vi "AdminLogInGetNoOfTrialsForOneStudent(SubVI).vi"(10 "Admin no":string, 11 "Refnum in":T1) -> (3 "NoOfTrials":i32)   [LabVIEW 2013]
uses:
  <vilib>/addons/database/Connection.llb/Conn ObjectReference.ctl
  <vilib>/addons/database/_DB Variant To Data/Database Variant To Data.xnode
  <vilib>/addons/database/NI_Database_API.lvlib
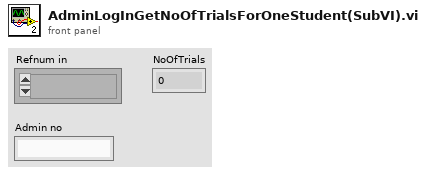
[diagram p1: front panel]
types:
  T1 = typedef "NI_Database_API.lvlib/Conn ObjectReference.ctl" = refnum<k1>
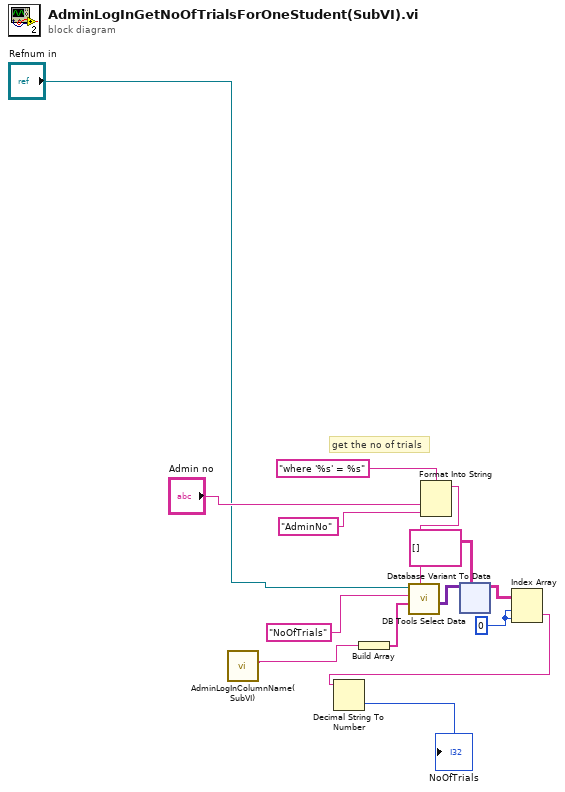
[diagram p0: block diagram]
diagram:
  w8 = 0 ("disabled index (col)")
  # "get the no of trials"
  n1 = call "AdminLogInColumnName(SubVI).vi"() -> ("Path for Score Table"=w1:string)  [unwired: 11 in]
  n2 = Build Array(w1) -> (w5:string[])
  n3 = Format Into String(format string="where '%s' = %s", "Admin no", "AdminNo") -> (resulting string=w2:string)  [unwired: 2 in, 1 out]
  n4 = call <vilib>:"DB Tools Select Data.vi"("condition"=w2, "columns"=w5, "table"="NoOfTrials", "connection reference"="Refnum in") -> ("data"=w9:variant[][])  [unwired: 2 in, 2 out]
  n5 = xnode "Database Variant To Data"("database variant"=w9, "type"=string[][] []) -> ("data"=w11:string[][])  [unwired: 1 in, 1 out]
  n6 = Index Array(array=w11, index (row)=w8, index (col)=w8) -> (element=w7:string)
  n7 = Decimal String To Number(string=w7) -> (number=→"NoOfTrials":i32)  [unwired: 2 in, 1 out]
